vi "Create Weather Forecast Graph Data.vi"(8 "error in (no error)":errorcluster, 11 "Weather Forecast Response":T1) -> (0 "error out":errorcluster, 3 "Weather Forecast Data":T2(graph))   [LabVIEW 2025, in "Weather Actor.lvlib" / "Weather.lvclass"]
uses:
  Weather.lvclass
  Weather.lvclass/Weather.ctl
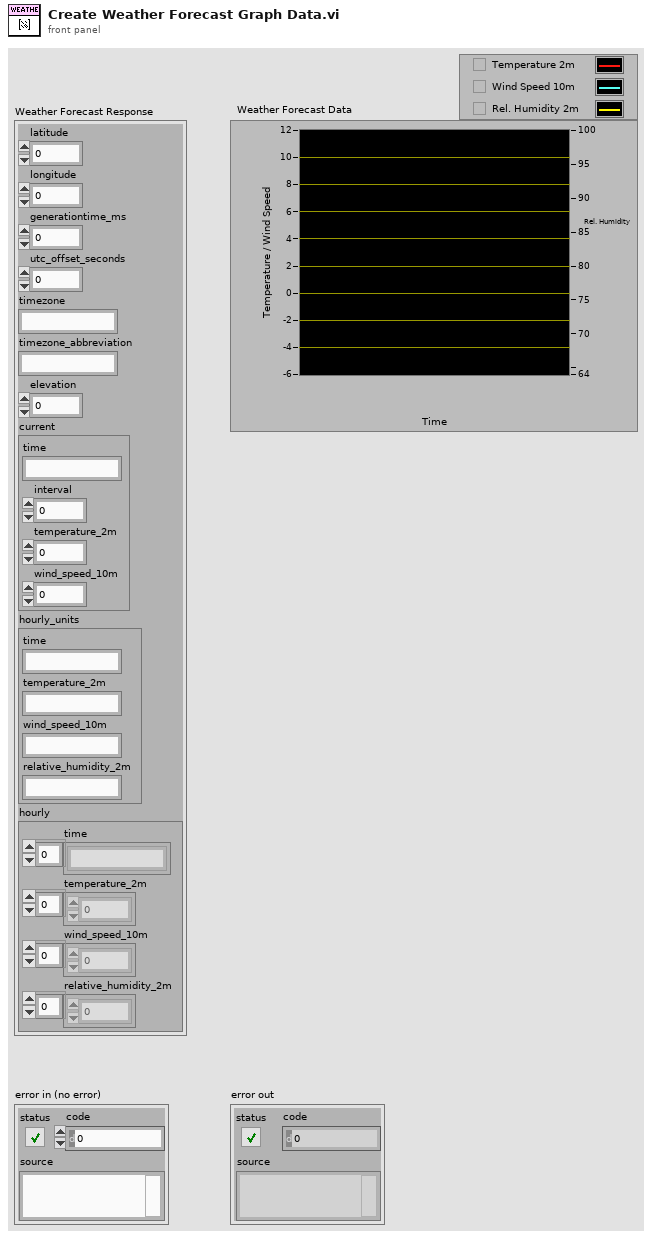
[diagram p1: front panel]
types:
  T1 = cluster{"latitude":dbl, "longitude":dbl, "generationtime_ms":dbl, "utc_offset_seconds":i32, "timezone":string, "timezone_abbreviation":string, "elevation":dbl, "current":cluster{"time":string, "interval":i32, "temperature_2m":dbl, "wind_speed_10m":dbl}, "hourly_units":cluster{"time":string, "temperature_2m":string, "wind_speed_10m":string, "relative_humidity_2m":string}, "hourly":cluster{"time":string[], "temperature_2m":dbl[], "wind_speed_10m":dbl[], "relative_humidity_2m":dbl[]}}
  T2 = cluster{timestamp[], "relative_humidity_2m":dbl[]}[]
  T3 = cluster{"X-Axis Time":timestamp[], "temperature_2m":dbl[]}
  T4 = cluster{"X-Axis Time":timestamp[], "wind_speed_10m":dbl[]}
  T5 = cluster{"X-Axis Time":timestamp[], "relative_humidity_2m":dbl[]}
  T6 = cluster{"X-Axis Time":timestamp[], "relative_humidity_2m":dbl[]}[]
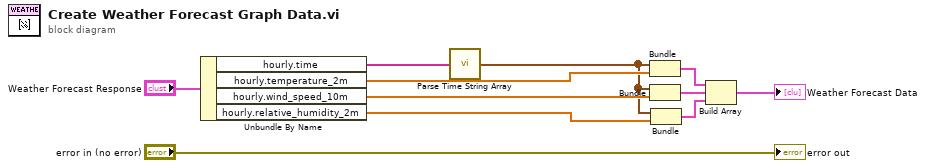
[diagram p0: block diagram]
diagram:
  n1 = Unbundle By Name("Weather Forecast Response") -> ("hourly.time"=w2:string[], "hourly.temperature_2m"=w11:dbl[], "hourly.wind_speed_10m"=w10:dbl[], "hourly.relative_humidity_2m"=w9:dbl[])
  n2 = call "Parse Time String Array.vi"("time"=w2) -> ("X-Axis Time"=w3:timestamp[])  [unwired: 4 in]
  n3 = Bundle("X-Axis Time"=w3, "temperature_2m"=w11) -> (w6:T3)  [unwired: 1 in]
  n4 = Bundle("X-Axis Time"=w3, "wind_speed_10m"=w10) -> (w8:T4)  [unwired: 1 in]
  n5 = Bundle("X-Axis Time"=w3, "relative_humidity_2m"=w9) -> (w7:T5)  [unwired: 1 in]
  n6 = Build Array(w6, w8, w7) -> (→"Weather Forecast Data":T6)
  "error out" <- "error in (no error)"
